vi "Program.vi"(8 "error in (no error)":errorcluster, 10 "Image":string, 11 "reference in":refnum<class "JTAG_Cyclone.lvclass">) -> (0 "error out":errorcluster, 1 "msg":string, 2 "Success":bool, 3 "reference in":refnum<class "JTAG_Cyclone.lvclass">)   [LabVIEW 2022 SP3, in "JTAG_Cyclone.lvlib" / "JTAG_Cyclone.lvclass"]
uses:
  JTAG_Cyclone.lvclass
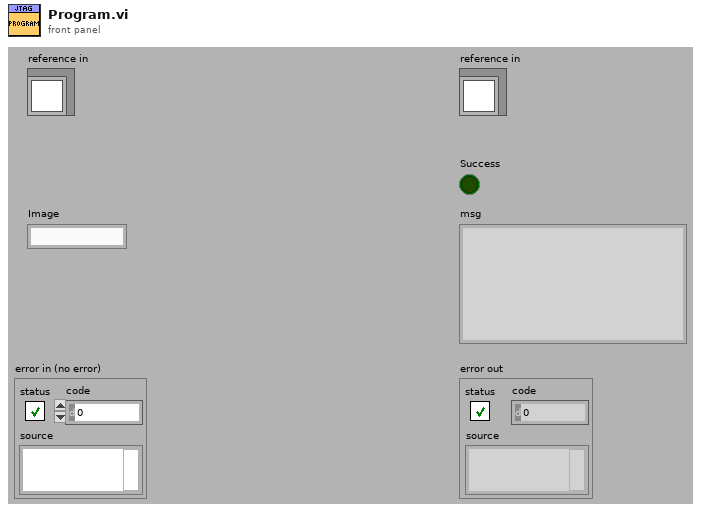
[diagram p1: front panel]
types:
  T1 = typedef "JTAG_Cyclone.lvlib/JTAG_Cyclone.lvclass/ObjectAttributes.ctl" = cluster{"Config":T2, "Success":bool, "Msg":string, "active image":string}
  T2 = typedef "JTAG_Cyclone.lvlib/JTAG_Cyclone.lvclass/Config.ctl" = cluster{"Cyclone_API_Path":path, "Cyclone_Name":string}
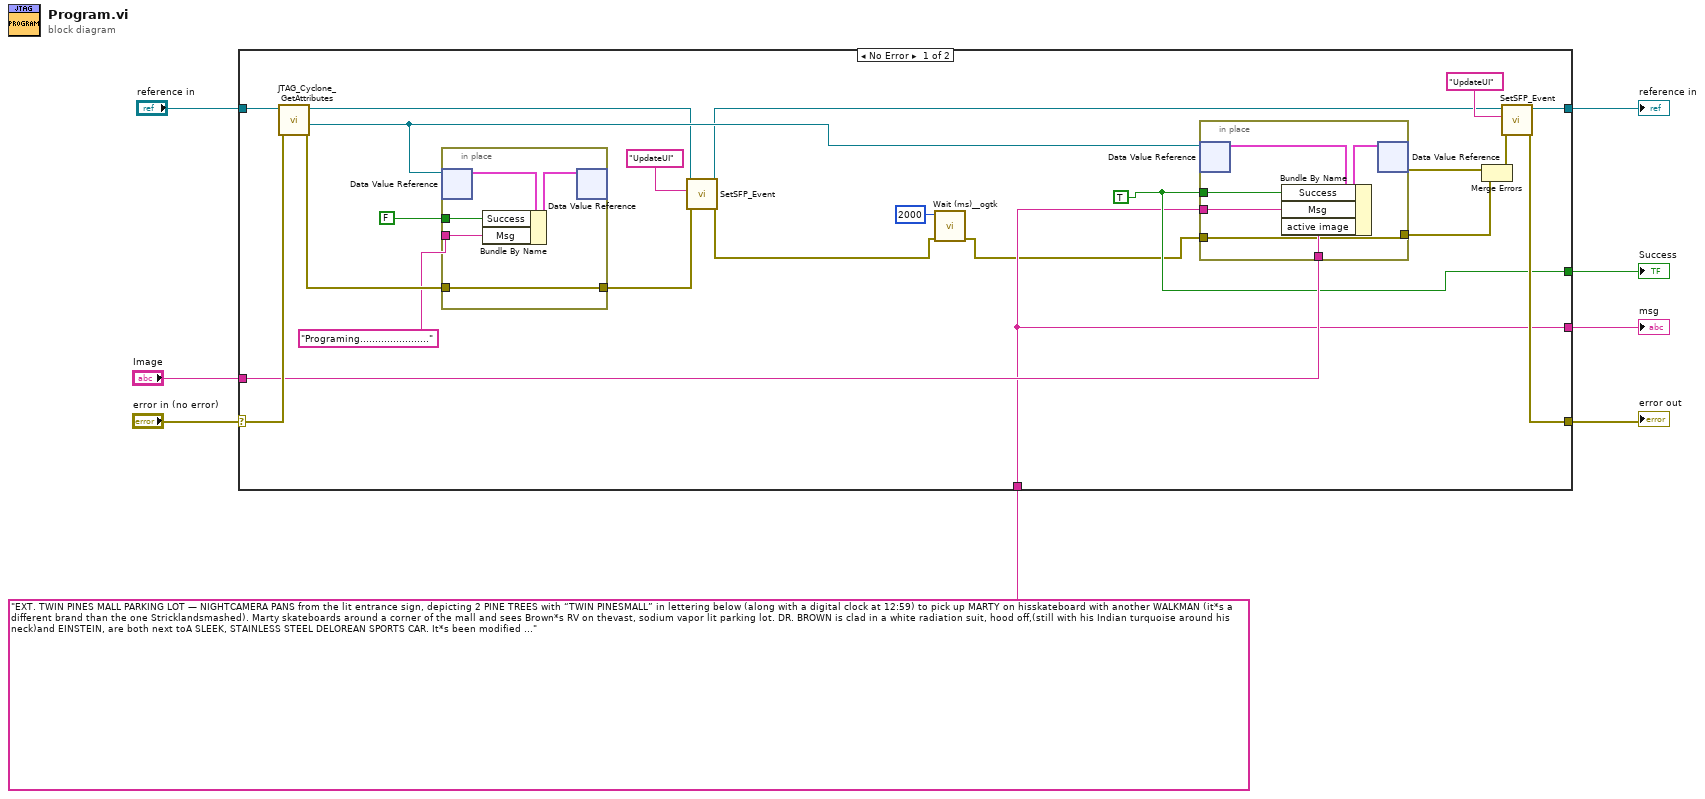
[diagram p0: block diagram]
diagram:
  n1 = case shown="No Error" "error in (no error)" {
    selector: "error in (no error)" -> [w30 w43]
    tunnel: [w27 w43] -> w7
    tunnel: [w28 w42] -> w5
    tunnel: "reference in" -> [w29 w42]
    tunnel: "Image" -> [w15 _]
    tunnel: "EXT. TWIN PINES MALL PARKING LOT — NIGHTCAMERA PANS from the lit entrance sign, depicting 2 PINE TREES with “TWIN PINESMALL” in lettering below (along with a digital clock at 12:59) to pick up MARTY on hisskateboard with another WALKMAN (it*s a different brand than the one Stricklandsmashed). Marty skateboards around a corner of the mall and sees Brown*s RV on thevast, sodium vapor lit parking lot. DR. BROWN is clad in a white radiation suit, hood off,(still with his Indian turquoise around his neck)and EINSTEIN, are both next toA SLEEK, STAINLESS STEEL DELOREAN SPORTS CAR. It*s been modified with somewicked looking units on its rear engine, giving it a particularly dangerous feel. There arecoils along the front and rear decks.There are also several small cases of supplies and equipment, and a piece of AmericanTourister luggage around the RV.Marty skateboards over, totally blown away by the car.MARTYJeez, Doc, a DeLorean! What the hell did you do to it?BROWNGrab the camera and start taping, Marty. I*ll explain as we go.Brown indicates a HOME VIDEO CAMERA nearby. Marty picks it up.MARTYAnd what*s with the Devo suit?Brown lifts open the driver*s side gull wing door.BROWNCome on, Einstein. Get in, boy.*16-A****17***\n18The dog obediently jumps in and sits in the driver*s seat. Brown buckles him in with theshoulder harness. The dog has a BATTERY OPERATED DIGITAL CLOCK hangingaround his neck.Marty begins taping, handheld, cinema verite style.BROWN(to Marty and video camera)All right, this is test #1. Please note that Einstein*s clock here is in precisesynchronization with my control watch.Brown holds up a digital watch next to Einstein*s clock; indeed, the two are in dead sync.BROWN(to the dog)Good luck, Einie.Brown reaches in and starts the ignition. The DeLorean engine ROARS to life. Brown turnson the headlights and lowers the gull wing door, sealing Einstein in.He steps back and picks up a REMOTE CONTROL UNIT, similar to one for a radiocontrolled toy car. There are buttons labeled “Accelerator” and “Brake”, a joystick, and anL.E.D. digital readout labeled “Miles Per Hour.” Brown flicks the power switch on and, usingthe accelerator button and joystick for steering, sends the DeLorean down to the far, farend of the parking lot. He turns the car around so that it*s pointing toward them, idling.BROWNHere we go, Marty. If my calculations are correct, when the car hits 88 milesan hour, you*re gonna see some serious shit.Brown takes a deep breath, then pushes the accelerator button.The DeLorean takes off, shifting gears automatically.The L.E.D. speedometer passes 30.The stainless steel vehicle zooms faster... past 40...Marty is getting it all on tape.Brown watches intently. The speedometer climbs past 60.IN THE CAR, Einstein remains calmly in the driver*s seat. Gauges and instrument lightsmounted behind him begin flashing.Brown*s finger holds the accelerator button down.The meter passes 75.The DeLorean keeps accelerating, approaching Marty and Brown. The coils mountedaround the car begin glowing.EXT. MALL, DELOREAN — NIGHTThe speedometer hits 85... 86... 87... 88...18\n192021The automobile is suddenly engulfed by a BLINDING WHITE GLOW — then, BLAM! It*sgone, a TRAIL OF FIRE left in its wake.Brown and Marty are hit by a sharp blast of air. Marty blinks in disbelief: it*s as if the carnever existed. Only the LICENSE PLATE is left behind — a vanity plate: “NO TIME.”BROWN(elated)What*d I tell you? 88 miles per hour! Temporal displacement occurred at(checks watch) exactly 1:02 a.m. and zero seconds.MARTY(shocked)Christ Almighty! You disintegrated Einstein!BROWNCalm down, Marty. I didn*t disintegrate anything. The molecular structure ofboth Einstein and the car are completely intact.MARTYThen where the hell are they?BROWNThe appropriate question is: WHEN the hell are they. You see, Einstein hasjust become the world*s first time traveler. I sent him into the future — oneminute into the future, to be exact. And at exactly 1:03 a.m. and zeroseconds, we shall catch up to him... and the time machine.MARTYTime machine? Are you trying to tell me you built a time machine out of aDeLorean?BROWN(smiles, modestly)The way I figured it, if you*re gonna build a time machine into a car, why notdo it with some style? Besides, the stainless steel construction made the fluxdispersal—(his digital watch BEEPS)Ten seconds! Roll tape — and brace yourself for a sudden displacement ofair.Marty aims the camera right where the DeLorean disappeared. Brown grips the remotecontrol unit tightly and counts down.BROWN5...4...3...2...1...Their hair stands up on end, charged up with static electricity..." -> [w13 _]
    tunnel: [w14 _] -> w2
    tunnel: [w13 _] -> w1
    frame No Error {
      w14 = TRUE ("Success")
      n2 = call "JTAG_Cyclone_GetAttributes.vi"("error in (no error)"=w30, "reference in"=w29) -> ("error out"=w21:errorcluster, "DataRef"=w22:refnum<data-value>, "reference out"=w17:refnum<class "JTAG_Cyclone.lvclass">)  [unwired: 6 in, 1 out]
      n3 = in-place {
        in-place-border: w21 -> [w33]
        in-place-border: [w33] -> w20
        in-place-border: FALSE -> [w32]
        in-place-border: "Programing......................." -> [w31]
        n4 = in-place-dvr #1(w22) -> (w35:T1)  [unwired: 1 out]
        n5 = Bundle By Name(cluster=w35, "Success"=w32, "Msg"=w31) -> (w34:T1)
        n6 = in-place-dvr #1(w34) -> ()  [unwired: 2 out]
      }
      n7 = call-dynamic "SetSFP_Event.vi"("error in (no error)"=w20, "msg"="UpdateUI", "reference in"=w17) -> ("error out"=w11:errorcluster, "reference out"=w16:refnum<class "JTAG_Cyclone.lvclass">)  [unwired: 7 in]
      n8 = call <userlib>:"Wait (ms)__ogtk.vi"("error in (no error)"=w11, "milliseconds to wait"=u32 2000) -> ("error out"=w10:errorcluster)  [unwired: 8 in, 1 out]
      n9 = in-place {
        in-place-border: w15 -> [w39]
        in-place-border: w13 -> [w38]
        in-place-border: w14 -> [w37]
        in-place-border: w10 -> [w36]
        in-place-border: [w36] -> w12
        n10 = in-place-dvr #2(w22) -> (w41:T1)  [unwired: 1 out]
        n11 = Bundle By Name(cluster=w41, "Success"=w37, "Msg"=w38, "active image"=w39) -> (w40:T1)
        n12 = in-place-dvr #2(w40) -> (w24:errorcluster)  [unwired: 1 out]
      }
      n13 = Merge Errors(w24, w12) -> (w23:errorcluster)
      n14 = call-dynamic "SetSFP_Event.vi"("error in (no error)"=w23, "msg"="UpdateUI", "reference in"=w16) -> ("error out"=w27:errorcluster, "reference out"=w28:refnum<class "JTAG_Cyclone.lvclass">)  [unwired: 7 in]
    }
    frame Error {
    }
  }
  "error out" <- w7
  "reference in" <- w5
  "Success" <- w2
  "msg" <- w1
